vi "ParallelLMS1.vi"() -> ()   [LabVIEW 2014]
uses:
  Hokuyo URG Series.lvlib
panel:
  out "Magnitude":dbl[](array[numeric])
  out "LMS Local Map":i32[][](array[numeric])
  in  "LMS Real/Sim":bool
  in  "LMS Com Port":refnum<visa-resource-name>
  in  "Stop?":bool
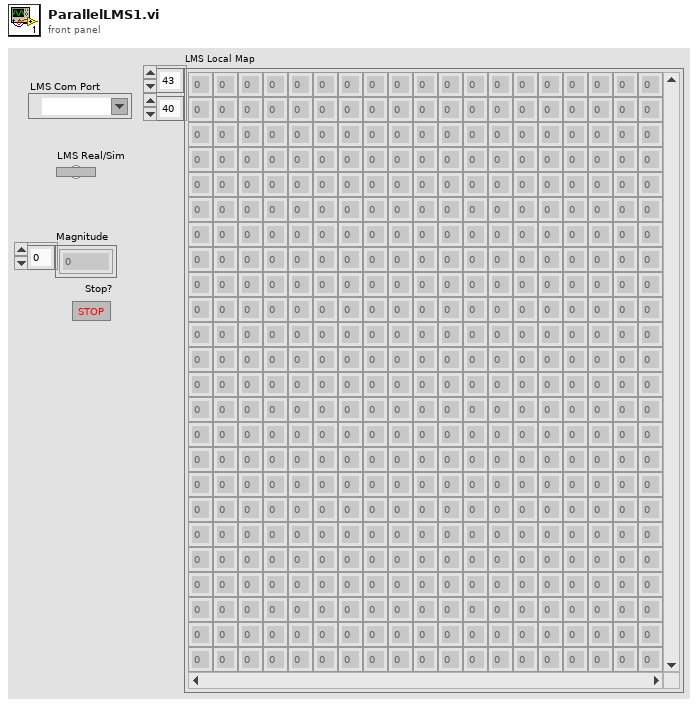
[diagram p1: front panel]
types:
  T1 = cluster{"LMS Com port":refnum<visa-resource-name>, "Error Out":errorcluster, "Real/Sim":bool, "First Run?":i32, "LMS Local Map ":dbl[][], "Magnitude":dbl[]}
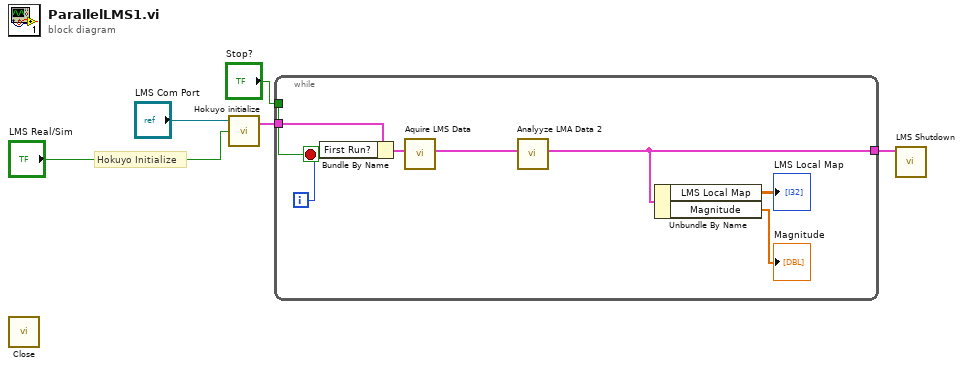
[diagram p0: block diagram]
diagram:
  # "Hokuyo Initialize"
  n1 = call "Close.vi"() -> ()  [unwired: 11 in, 1 out]
  n2 = call "Hokuyo initialize.vi"("real/sim"="LMS Real/Sim", "Hokuyo Port"="LMS Com Port") -> ("LMS Information Cluster"=w5:T1)  [unwired: 2 in]
  n3 = while {
    tunnel: w5 -> [w12]
    tunnel: "Stop?" -> [w9]
    tunnel: [w6] -> w1
    i -> [w11]
    stop <- w9 stop-if-true
    n4 = Bundle By Name(cluster=w12, "First Run?"=w11) -> (w10:T1)
    n5 = call "Aquire LMS Data.vi"("LMS Information Cluster In"=w10) -> ("LMS Information Cluster Out"=w13:T1)  [unwired: 10 in]
    n6 = call "Analyyze LMA Data 2.vi"("LMS Information Cluster In"=w13) -> ("LMS Information Cluster Out"=w6:T1)  [unwired: 10 in]
    n7 = Unbundle By Name(w6) -> ("LMS Local Map"=→"LMS Local Map":dbl[][], "Magnitude"=→"Magnitude":dbl[])
  }
  n8 = call "LMS Shutdown.vi"("LMS Information Cluster In"=w1) -> ()  [unwired: 11 in]
